vi "FlatToRichnixnet_grpc_LinDiagnosticScheduleChangeRequest.vi"(5 "OutputClusterType":T1, 11 "InputCluster":T2) -> (3 "OutputCluster":T1)   [LabVIEW 2025, in "xnet-grpc_client.lvlib"]
uses:
  nixnet_grpc_LinDiagnosticScheduleChangeRequest_Flat.ctl
  nixnet_grpc_LinDiagnosticSchedule.ctl
  nixnet_grpc_LinDiagnosticScheduleChangeRequest.ctl
  nixnet_grpc_LinDiagnosticScheduleChangeRequest_schedule_enum/nixnet_grpc_LinDiagnosticScheduleChangeRequest_schedule_enum.lvclass
  xnet-grpc_client.lvlib
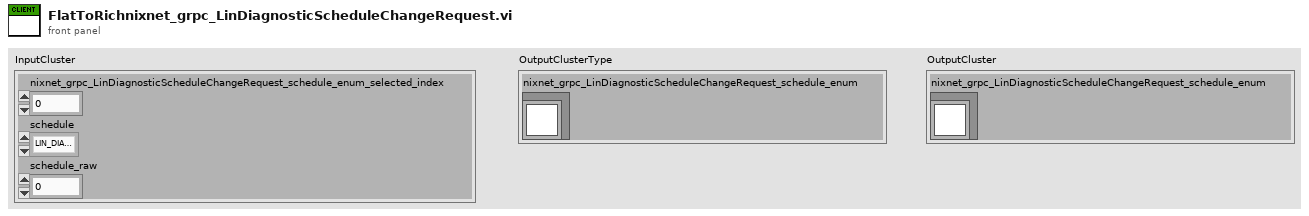
[diagram p1: front panel]
types:
  T1 = typedef "xnet-grpc_client.lvlib/nixnet_grpc_LinDiagnosticScheduleChangeRequest.ctl" = cluster{"nixnet_grpc_LinDiagnosticScheduleChangeRequest_schedule_enum":refnum<class "nixnet_grpc_LinDiagnosticScheduleChangeRequest_schedule_enum.lvclass">}
  T2 = typedef "xnet-grpc_client.lvlib/nixnet_grpc_LinDiagnosticScheduleChangeRequest_Flat.ctl" = cluster{"nixnet_grpc_LinDiagnosticScheduleChangeRequest_schedule_enum_selected_index":i32, "schedule":T3, "schedule_raw":u32}
  T3 = typedef "xnet-grpc_client.lvlib/nixnet_grpc_LinDiagnosticSchedule.ctl" = enum32{"LIN_DIAGNOSTIC_SCHEDULE_NULL", "LIN_DIAGNOSTIC_SCHEDULE_MASTER_REQ", "LIN_DIAGNOSTIC_SCHEDULE_SLAVE_RESP"}
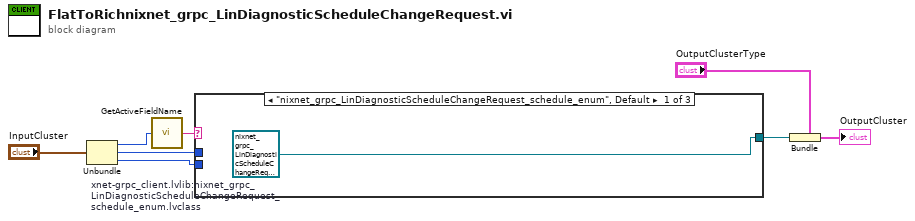
[diagram p0: block diagram]
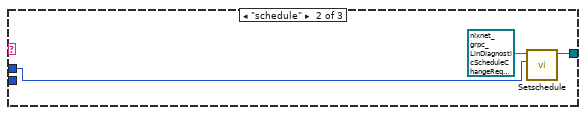
[diagram p2: hidden frame]
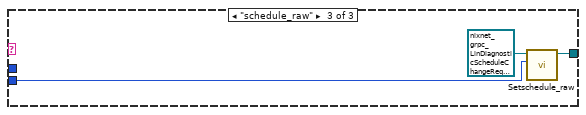
[diagram p3: hidden frame]
diagram:
  n1 = Unbundle "Unbundle"("InputCluster") -> ("nixnet_grpc_LinDiagnosticScheduleChangeRequest_schedule_enum_selected_index"=w5:i32, "schedule"=w2:T3, "schedule_raw"=w1:u32)
  n2 = call "GetActiveFieldName.vi"("protobuf index"=w5) -> ("oneof field name"=w4:string)
  n3 = case "nixnet_grpc_LinDiagnosticScheduleChangeRequest_schedule_enum" shown="\"nixnet_grpc_LinDiagnosticScheduleChangeRequest_schedule_enum\", Default" w4 {
    tunnel: [w9 w11 w14] -> w3
    tunnel: w2 -> [_ w12 _]
    tunnel: w1 -> [_ _ w15]
    frame "nixnet_grpc_LinDiagnosticScheduleChangeRequest_schedule_enum", Default {
      w9 = refnum<class "nixnet_grpc_LinDiagnosticScheduleChangeRequest_schedule_enum.lvclass"> refnum  # xnet-grpc_client.lvlib:nixnet_grpc_LinDiagnosticScheduleChangeRequest_schedule_enum.lvclass
    }
    frame "schedule" {
      n4 = call "Setschedule.vi"("Set_Val"=w12, "OneOfTemplate in"=refnum<class "nixnet_grpc_LinDiagnosticScheduleChangeRequest_schedule_enum.lvclass"> refnum) -> ("OneOfTemplate out"=w11:refnum<class "nixnet_grpc_LinDiagnosticScheduleChangeRequest_schedule_enum.lvclass">)  [unwired: 8 in, 1 out]
    }
    frame "schedule_raw" {
      n5 = call "Setschedule_raw.vi"("Set_Val"=w15, "OneOfTemplate in"=refnum<class "nixnet_grpc_LinDiagnosticScheduleChangeRequest_schedule_enum.lvclass"> refnum) -> ("OneOfTemplate out"=w14:refnum<class "nixnet_grpc_LinDiagnosticScheduleChangeRequest_schedule_enum.lvclass">)  [unwired: 8 in, 1 out]
    }
  }
  n6 = Bundle "Bundle"(cluster="OutputClusterType", "nixnet_grpc_LinDiagnosticScheduleChangeRequest_schedule_enum"=w3) -> (→"OutputCluster":T1)
